vi "FT_sensor_tester old.vi"() -> ()   [LabVIEW 2018]
uses:
  <vilib>/Analysis/baseanly.llb/A x Vector.vi
  <vilib>/Analysis/NI_AALBase.lvlib
panel:
  out "Array":T1(array[cluster])
  out "x-y":u16
  out "Calibrated":dbl[](array[numeric]) format="%.2f"
  in  "Stop Acquisition":bool
  in  "Start Acquisition":bool
  in  "Get Sensor Buffer":bool
  out "Sensor Data":T2
  out "System Status":cluster{"boardState":u8}
  in  "Get Sensor Data":bool
  out "Error Code":T3(ring)
  out "Return FID":u8=2
  out "FID":u8=2
  in  "IP Address":string="192.168.5.001"
  out "System Info":T4
  out "error out":errorcluster
  in  "Get System Info":bool
  in  "Get System Status":bool
  in  "Stop":bool
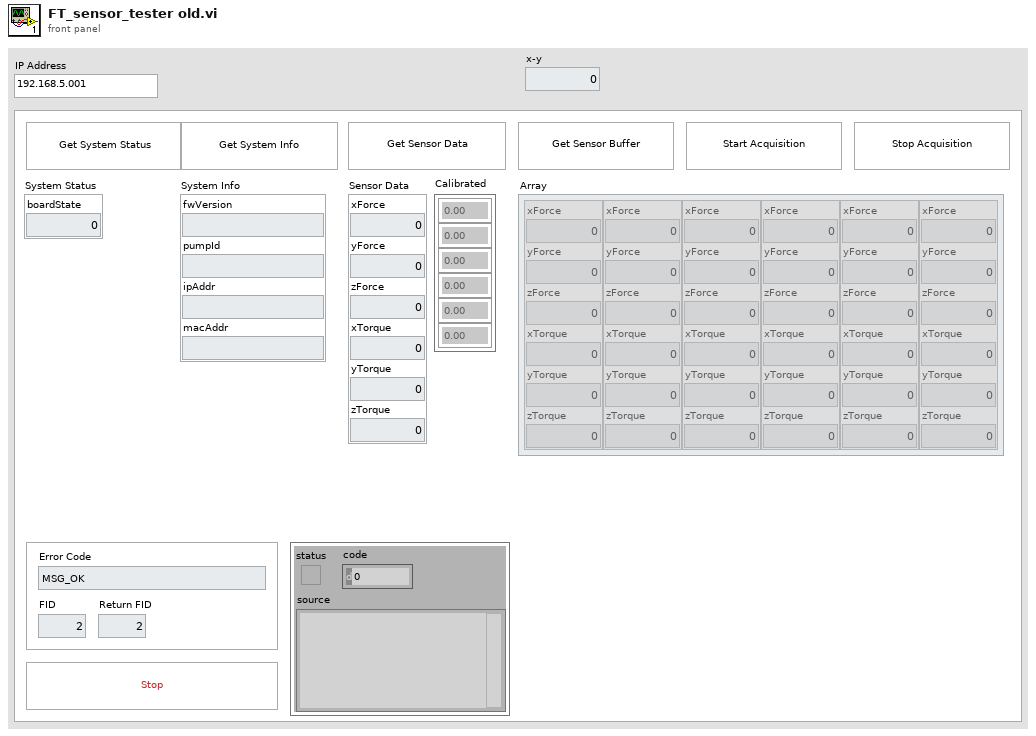
[diagram p1: front panel]
types:
  T1 = cluster{"xForce":sgl, "yForce":sgl, "zForce":sgl, "xTorque":sgl, "yTorque":sgl, "zTorque":sgl}[]
  T2 = cluster{"xForce":sgl, "yForce":sgl, "zForce":sgl, "xTorque":sgl, "yTorque":sgl, "zTorque":sgl}
  T3 = enum8{"MSG_OK", "MSG_ERROR_NOT_SUPPORTED", "MSG_ERROR_SENSOR_DISCONNECTED", "MSG_ERROR_READING_PENDING"}
  T4 = cluster{"fwVersion":string, "pumpId":string, "ipAddr":string, "macAddr":string}
  T5 = cluster{"fwVersion":string, "pumpId":string, "macAddr":string, "ipAddr":string}
  T6 = enum16{"big-endian, network order", "native, host order", "little-endian"}
  T7 = cluster{"pumpState":i32, "suppliedVolume_ml":sgl, "flowRate_mlmin":sgl, "home":i32, "port":i32}
  T8 = cluster{"connection ID":refnum<k5>, "header length":u16}
  T9 = cluster{"boardState":u8, "tempSetpoint":sgl, "pH connected":bool, "Temp connected":bool, "pidOutput":dbl, "pidIntegral":dbl, "pidSetpoint":sgl, "pidStep":sgl, "pidMethod":u8}
  T10 = cluster{"header":cluster{"length":u16, "fid":u8, "error":u8}}
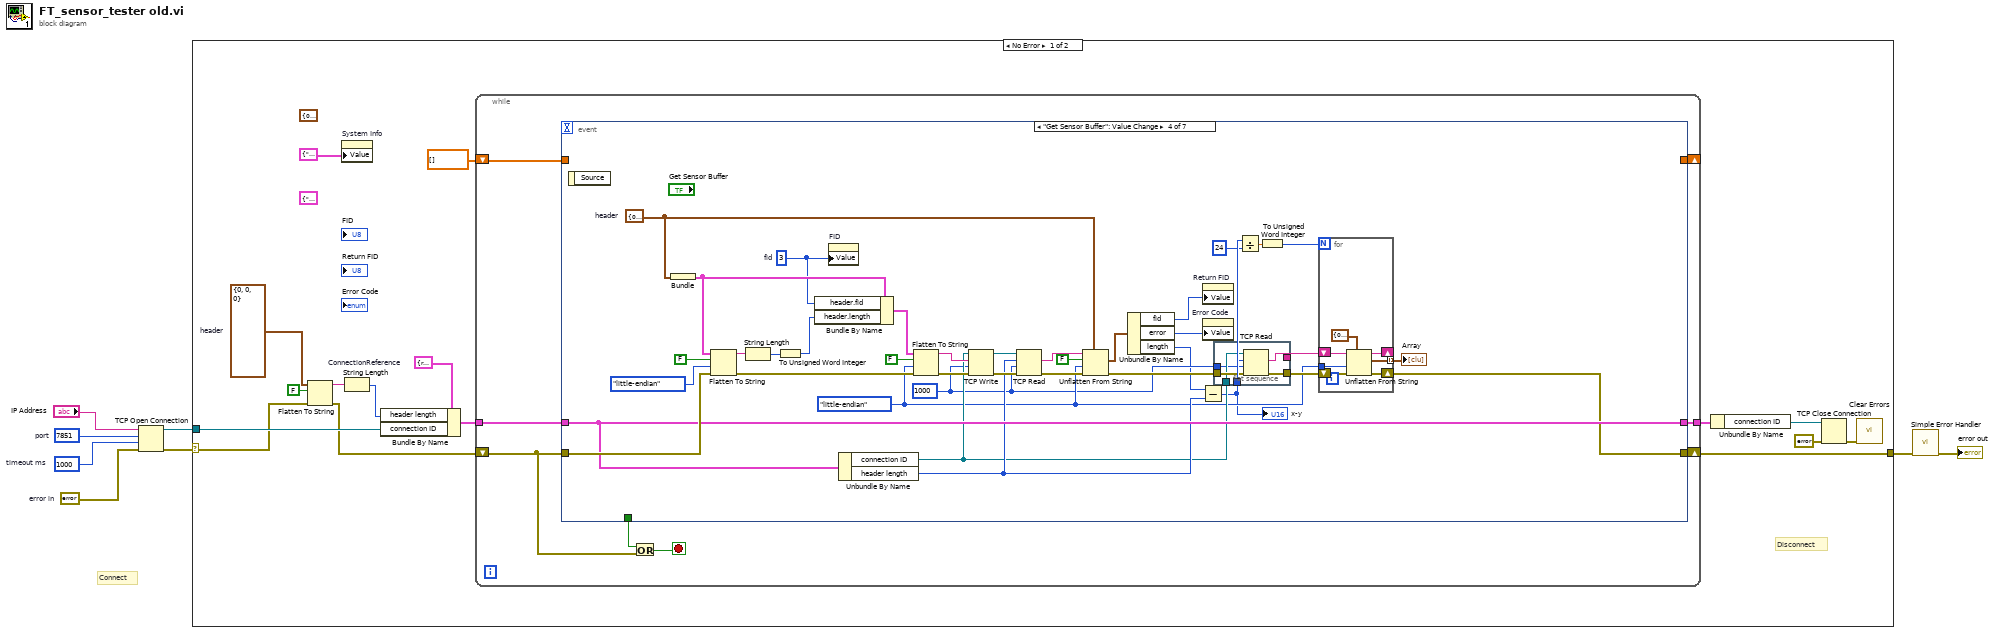
[diagram p0: block diagram]
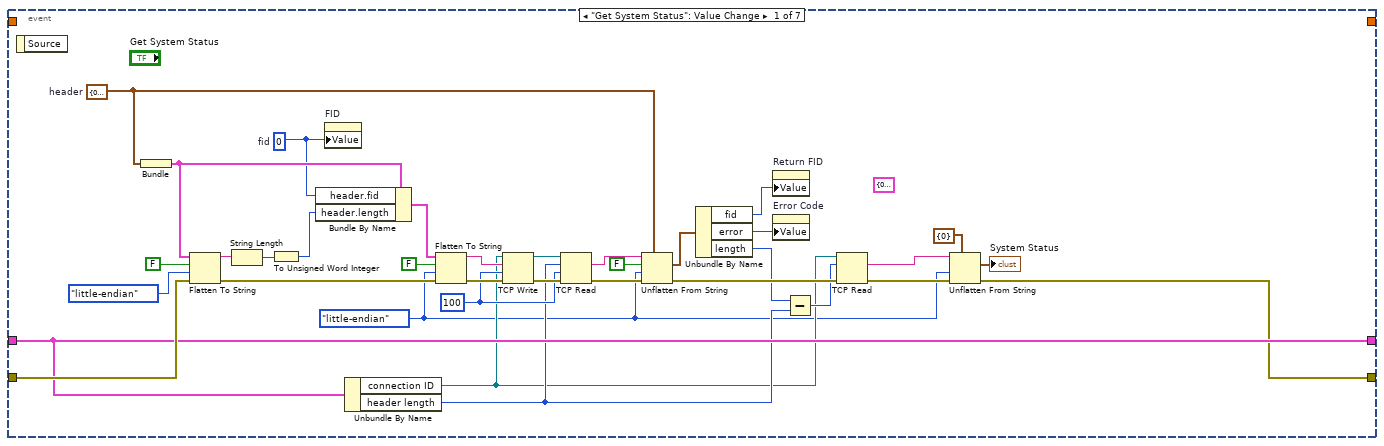
[diagram p2: hidden frame]
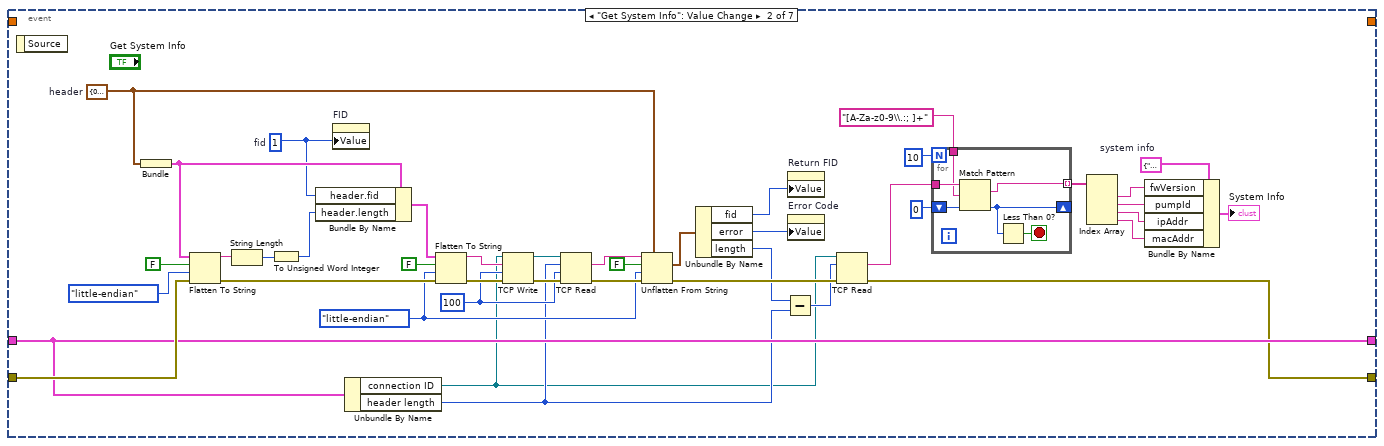
[diagram p3: hidden frame]
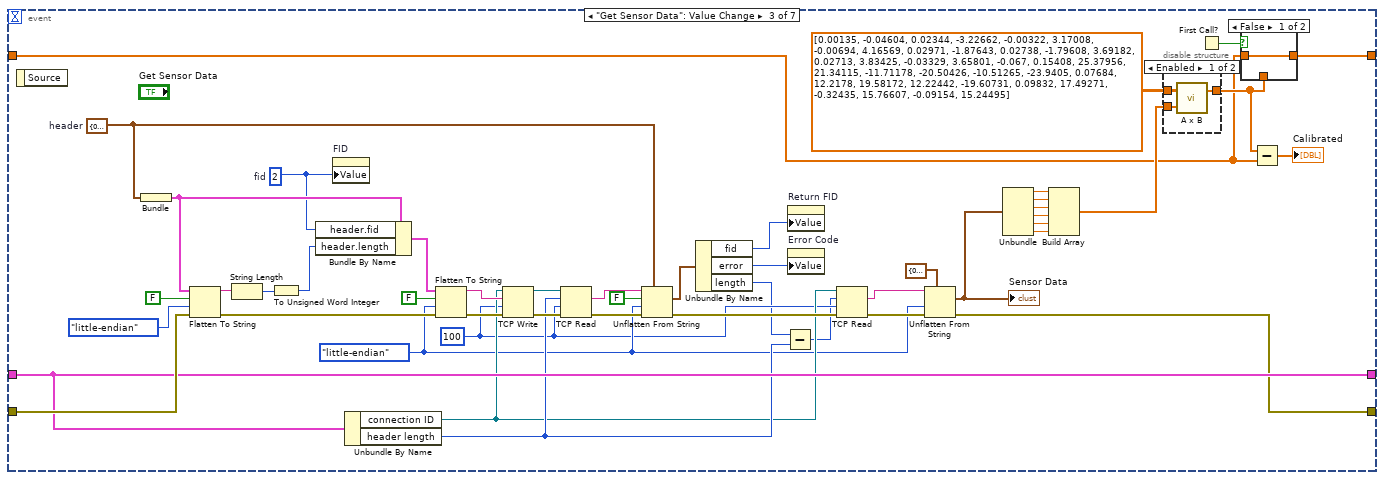
[diagram p4: hidden frame]
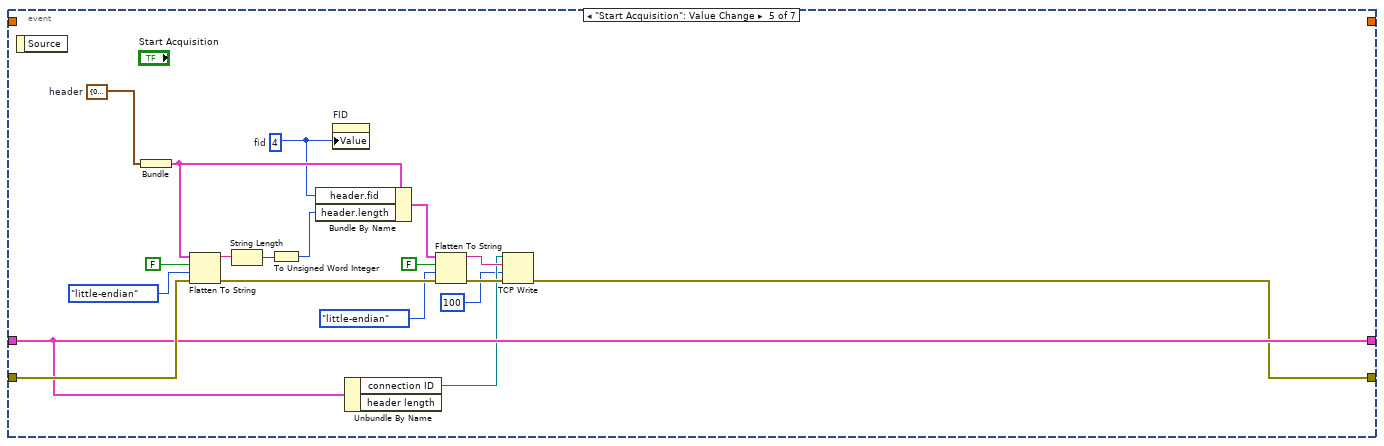
[diagram p7: hidden frame]
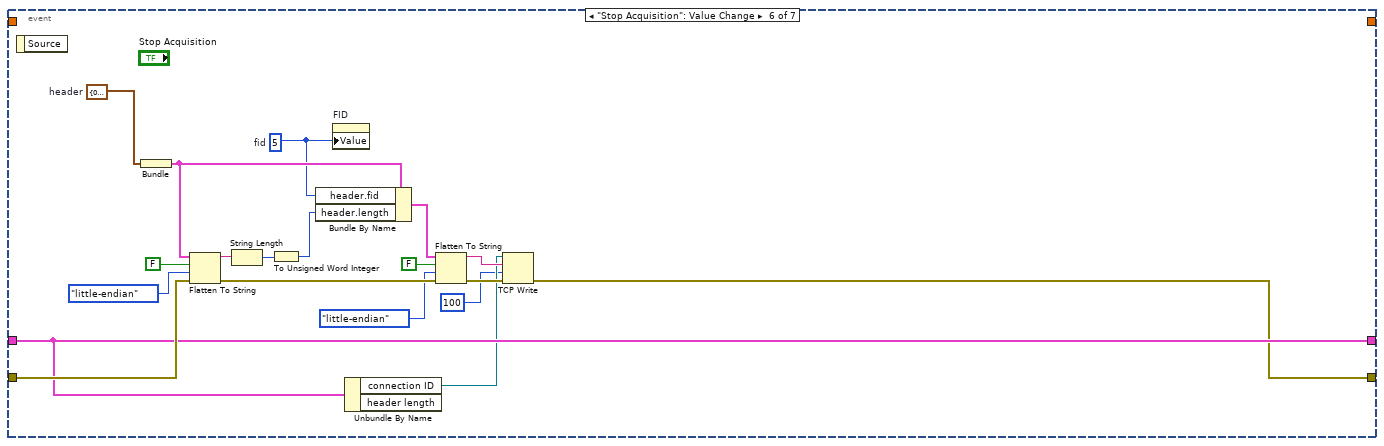
[diagram p8: hidden frame]
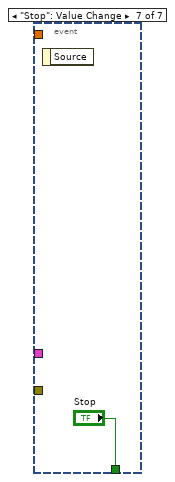
[diagram p9: hidden frame]
diagram:
  w6 = errorcluster {"status"=FALSE, "code"=0, "source"=""}  # error in
  w7 = 1000  # timeout ms
  w8 = u16 7851  # port
  # "Connect"
  n1 = TCP Open Connection(address="IP Address", remote port or service name=w8, timeout ms (60000)=w7, error in (no error)=w6) -> (connection ID=w5:refnum<k5>, error out=w1:errorcluster)  [unwired: 1 in]
  n2 = case shown="No Error" w1 {
    selector: w1 -> [w11 w259]
    tunnel: w5 -> [w20 _]
    tunnel: [w12 w259] -> w2
    frame No Error {
      (unwired) cluster{"axis":string, "stepPeriod (ms)":string} {"axis"="", "stepPeriod (ms)"=""} ("Return Motor Config")
      (unwired) T7 {"pumpState"=0, "suppliedVolume_ml"=0.0, "flowRate_mlmin"=0.0, "home"=0, "port"=0} ("Status")
      w19 = cluster{"length":u16, "fid":u8, "error":u8} {"length"=0, "fid"=0, "error"=0}  # header
      w21 = T8 {"connection ID"=refnum, "header length"=0}  # ConnectionReference
      # "Disconnect"
      n3 = Flatten To String(anything=w19, prepend array or string size? (T)=FALSE, error in (no error)=w11) -> (data string=w17:string, error out=w13:errorcluster)  [unwired: 1 in, 1 out]
      n4 = property on="System Info" class="Clust (strict)"("Value"=T5 {"fwVersion"="", "pumpId"="", "macAddr"="", "ipAddr"=""} ("system info")) -> ()  [unwired: 2 in, 2 out]
      n5 = String Length(string=w17) -> (length=w16:i32)
      n6 = Bundle By Name(cluster=w21, "header length"=w16, "connection ID"=w20) -> (w15:T8)
      n7 = while {
        tunnel: w15 -> [w32]
        tunnel: [w31] -> w14
        shift-right: [w30] -> w12
        shift-left: w13 -> [w28]
        shift-right: [w26] -> _
        shift-left: dbl[] [] ("A x Vector") -> [w25]
        stop <- w29 stop-if-true
        n8 = event shown="[3] \"Get Sensor Buffer\": Value Change" {
          selector: _ -> [_ _ _ _ _ _ _]
          dyn-events: _ -> [_ _ _ _ _ _ _]
          timeout: _ -> [_ _ _ _ _ _ _]
          tunnel: w32 -> [w56 w98 w152 w195 w227 w246 _]
          tunnel: [w56 w98 w152 w195 w227 w246 _] -> w31
          tunnel: w28 -> [w57 w99 w153 w196 w228 w247 _]
          tunnel: [w39 w75 w136 w179 w220 w239 _] -> w30
          tunnel: [_ _ _ _ _ _ "Stop"] -> w27
          tunnel: [_ _ w119 _ _ _ _] -> w26
          tunnel: w25 -> [_ _ w117 _ _ _ _]
          event "Get System Status": Value Change {
            (unwired) T9 {"boardState"=0, "tempSetpoint"=0.0, "pH connected"=FALSE, "Temp connected"=FALSE, "pidOutput"=0.0, "pidIntegral"=0.0, "pidSetpoint"=0.0, "pidStep"=0.0, "pidMethod"=0} ("Status")
            w48 = cluster{"length":u16, "fid":u8, "error":u8} {"length"=0, "fid"=0, "error"=0}  # header
            w50 = 100 ("timeout ms (25000)")
            w36 = u8 0  # fid
            w38 = T6."little-endian" ("byte order (0:big-endian, network order)")
            n9 = event-data() -> ()  [unwired: 1 in, 1 out]
            n10 = Bundle("header"=w48) -> (w63:T10)  [unwired: 1 in]
            n11 = Flatten To String(anything=w63, prepend array or string size? (T)=FALSE, byte order (0:big-endian, network order)=T6."little-endian", error in (no error)=w57) -> (data string=w61:string, error out=w62:errorcluster)  [unwired: 1 out]
            n12 = String Length(string=w61) -> (length=w60:i32)
            n13 = To Unsigned Word Integer(number=w60) -> (unsigned 16bit integer=w59:u16)
            n14 = Bundle By Name(cluster=w63, "header.fid"=w36, "header.length"=w59) -> (w64:T10)
            n15 = property on="FID" class="DigNum (strict)"("Value"=w36) -> ()  [unwired: 2 in, 2 out]
            n16 = Unbundle By Name(w56) -> ("connection ID"=w42:refnum<k5>, "header length"=w44:u16)
            n17 = Flatten To String(anything=w64, prepend array or string size? (T)=FALSE, byte order (0:big-endian, network order)=w38, error in (no error)=w62) -> (data string=w66:string, error out=w67:errorcluster)  [unwired: 1 out]
            n18 = TCP Write(connection ID=w42, data in=w66, error in (no error)=w67, 9:w50) -> (connection ID out=w51:refnum<k5>, error out=w52:errorcluster)  [unwired: 1 out]
            n19 = TCP Read(connection ID=w51, bytes to read=w44, error in (no error)=w52, 9:w50) -> (data out=w53:string, error out=w54:errorcluster)  [unwired: 1 in, 1 out]
            n20 = Unflatten From String(type=w48, binary string=w53, data includes array or string size? (T)=FALSE, byte order (0:big-endian, network order)=w38, error in (no error)=w54) -> (value=w49:cluster{"length":u16, "fid":u8, "error":u8}, error out=w46:errorcluster)  [unwired: 1 out]
            n21 = Unbundle By Name(w49) -> ("fid"=w37:u8, "error"=w35:u8, "length"=w45:u16)
            n22 = property on="Return FID" class="DigNum (strict)"("Value"=w37) -> ()  [unwired: 2 in, 2 out]
            n23 = property on="Error Code" class="Enum (strict)"("Value"=w35) -> ()  [unwired: 2 in, 2 out]
            n24 = Subtract(x=w45, y=w44) -> (x-y=w43:u16)
            n25 = TCP Read(connection ID=w42, bytes to read=w43, error in (no error)=w46) -> (data out=w41:string, error out=w40:errorcluster)  [unwired: 2 in, 1 out]
            n26 = Unflatten From String(type=cluster{"boardState":u8} {"boardState"=0} ("System Status"), binary string=w41, byte order (0:big-endian, network order)=w38, error in (no error)=w40) -> (value=→"System Status":cluster{"boardState":u8}, error out=w39:errorcluster)  [unwired: 1 in, 1 out]
          }
          event "Get System Info": Value Change {
            w87 = T4 {"fwVersion"="", "pumpId"="", "ipAddr"="", "macAddr"=""}  # system info
            w89 = cluster{"length":u16, "fid":u8, "error":u8} {"length"=0, "fid"=0, "error"=0}  # header
            w92 = 100 ("timeout ms (25000)")
            w70 = u8 1  # fid
            w91 = T6."little-endian" ("byte order (0:big-endian, network order)")
            n27 = event-data() -> ()  [unwired: 1 in, 1 out]
            n28 = Bundle("header"=w89) -> (w105:T10)  [unwired: 1 in]
            n29 = Flatten To String(anything=w105, prepend array or string size? (T)=FALSE, byte order (0:big-endian, network order)=T6."little-endian", error in (no error)=w99) -> (data string=w103:string, error out=w104:errorcluster)  [unwired: 1 out]
            n30 = String Length(string=w103) -> (length=w102:i32)
            n31 = To Unsigned Word Integer(number=w102) -> (unsigned 16bit integer=w101:u16)
            n32 = Bundle By Name(cluster=w105, "header.fid"=w70, "header.length"=w101) -> (w106:T10)
            n33 = property on="FID" class="DigNum (strict)"("Value"=w70) -> ()  [unwired: 2 in, 2 out]
            n34 = Unbundle By Name(w98) -> ("connection ID"=w71:refnum<k5>, "header length"=w73:u16)
            n35 = Flatten To String(anything=w106, prepend array or string size? (T)=FALSE, byte order (0:big-endian, network order)=w91, error in (no error)=w104) -> (data string=w108:string, error out=w109:errorcluster)  [unwired: 1 out]
            n36 = TCP Write(connection ID=w71, data in=w108, error in (no error)=w109, 9:w92) -> (connection ID out=w93:refnum<k5>, error out=w94:errorcluster)  [unwired: 1 out]
            n37 = TCP Read(connection ID=w93, bytes to read=w73, error in (no error)=w94, 9:w92) -> (data out=w95:string, error out=w96:errorcluster)  [unwired: 1 in, 1 out]
            n38 = Unflatten From String(type=w89, binary string=w95, data includes array or string size? (T)=FALSE, byte order (0:big-endian, network order)=w91, error in (no error)=w96) -> (value=w90:cluster{"length":u16, "fid":u8, "error":u8}, error out=w77:errorcluster)  [unwired: 1 out]
            n39 = Unbundle By Name(w90) -> ("fid"=w69:u8, "error"=w68:u8, "length"=w74:u16)
            n40 = Subtract(x=w74, y=w73) -> (x-y=w72:u16)
            n41 = property on="Return FID" class="DigNum (strict)"("Value"=w69) -> ()  [unwired: 2 in, 2 out]
            n42 = property on="Error Code" class="Enum (strict)"("Value"=w68) -> ()  [unwired: 2 in, 2 out]
            n43 = TCP Read(connection ID=w71, bytes to read=w72, error in (no error)=w77) -> (data out=w85:string, error out=w75:errorcluster)  [unwired: 2 in, 1 out]
            n44 = for {
              N: 10 -> [_]
              shift-right: [w111] -> _
              shift-left: 0 ("offset past match") -> [w115]
              tunnel: w85 -> [w114]
              tunnel: "[A-Za-z0-9\\.:; ]+" ("regular expression") -> [w113]
              tunnel: [w110] -> w82 mode=indexing
              stop <- w112 stop-if-true
              n45 = Match Pattern(string=w114, regular expression=w113, offset (0)=w115) -> (match substring=w110:string, offset past match=w111:i32)  [unwired: 2 out]
              n46 = Less Than 0?(x=w111) -> (x < 0?=w112:bool)
            }
            n47 = Index Array(array=w82) -> (element #1=w81:string, element #2=w80:string, element #3=w79:string, element #4=w78:string)  [unwired: 4 in]
            n48 = Bundle By Name(cluster=w87, "fwVersion"=w81, "pumpId"=w80, "ipAddr"=w79, "macAddr"=w78) -> (→"System Info":T4)
          }
          event "Get Sensor Data": Value Change {
            w145 = cluster{"length":u16, "fid":u8, "error":u8} {"length"=0, "fid"=0, "error"=0}  # header
            w133 = 100 ("timeout ms (25000)")
            w140 = u8 2  # fid
            w134 = T6."little-endian" ("byte order (0:big-endian, network order)")
            n49 = event-data() -> ()  [unwired: 1 in, 1 out]
            n50 = Bundle("header"=w145) -> (w159:T10)  [unwired: 1 in]
            n51 = Flatten To String(anything=w159, prepend array or string size? (T)=FALSE, byte order (0:big-endian, network order)=T6."little-endian", error in (no error)=w153) -> (data string=w157:string, error out=w158:errorcluster)  [unwired: 1 out]
            n52 = String Length(string=w157) -> (length=w156:i32)
            n53 = To Unsigned Word Integer(number=w156) -> (unsigned 16bit integer=w155:u16)
            n54 = Bundle By Name(cluster=w159, "header.fid"=w140, "header.length"=w155) -> (w160:T10)
            n55 = property on="FID" class="DigNum (strict)"("Value"=w140) -> ()  [unwired: 2 in, 2 out]
            n56 = Unbundle By Name(w152) -> ("connection ID"=w141:refnum<k5>, "header length"=w142:u16)
            n57 = Flatten To String(anything=w160, prepend array or string size? (T)=FALSE, byte order (0:big-endian, network order)=w134, error in (no error)=w158) -> (data string=w162:string, error out=w163:errorcluster)  [unwired: 1 out]
            n58 = TCP Write(connection ID=w141, data in=w162, error in (no error)=w163, 9:w133) -> (connection ID out=w147:refnum<k5>, error out=w148:errorcluster)  [unwired: 1 out]
            n59 = TCP Read(connection ID=w147, bytes to read=w142, error in (no error)=w148, 9:w133) -> (data out=w149:string, error out=w150:errorcluster)  [unwired: 1 in, 1 out]
            n60 = Unflatten From String(type=w145, binary string=w149, data includes array or string size? (T)=FALSE, byte order (0:big-endian, network order)=w134, error in (no error)=w150) -> (value=w146:cluster{"length":u16, "fid":u8, "error":u8}, error out=w143:errorcluster)  [unwired: 1 out]
            n61 = Unbundle By Name(w146) -> ("fid"=w139:u8, "error"=w138:u8, "length"=w130:u16)
            n62 = Subtract(x=w130, y=w142) -> (x-y=w131:u16)
            n63 = property on="Return FID" class="DigNum (strict)"("Value"=w139) -> ()  [unwired: 2 in, 2 out]
            n64 = property on="Error Code" class="Enum (strict)"("Value"=w138) -> ()  [unwired: 2 in, 2 out]
            n65 = TCP Read(connection ID=w141, bytes to read=w131, error in (no error)=w143, 9:w133) -> (data out=w135:string, error out=w137:errorcluster)  [unwired: 1 in, 1 out]
            n66 = Unflatten From String(type=T2 {"xForce"=0.0, "yForce"=0.0, "zForce"=0.0, "xTorque"=0.0, "yTorque"=0.0, "zTorque"=0.0} ("Sensor Data"), binary string=w135, byte order (0:big-endian, network order)=w134, error in (no error)=w137) -> (value=w128:T2, error out=w136:errorcluster)  [unwired: 1 in, 1 out]
            "Sensor Data" <- w128
            n67 = Unbundle(w128) -> ("xForce"=w127:sgl, "yForce"=w122:sgl, "zForce"=w123:sgl, "xTorque"=w124:sgl, "yTorque"=w125:sgl, "zTorque"=w126:sgl)
            n68 = Build Array(w127, w122, w123, w124, w125, w126) -> (w121:sgl[])
            n69 = disable-structure shown="Enabled" {
              disable-tunnel: dbl[][] [[0.00135, -0.04604, 0.02344, -3.22662, -0.00322, 3.17008], [-0.00694, 4.16569, 0.02971, -1.87643, 0.02738, -1.79608], [3.69182, 0.02713, 3.83425, -0.03329, 3.65801, -0.067], [0.15408, 25.37956, 21.34115, -11.71178, -20.50426, -10.51265], [-23.9405, 0.07684, 12.2178, 19.58172, 12.22442, -19.60731], [0.09832, 17.49271, -0.32435, 15.76607, -0.09154, 15.24495]] ("Calibration Matrix") -> [w166 _]
              disable-tunnel: w121 -> [w165 w167]
              disable-tunnel: [w164 w167] -> w118
              frame Enabled {
                n70 = call-poly <vilib>:"A x B.vi"("Vector"=w165, "A"=w166) -> ("A x Vector"=w164:dbl[])  [unwired: 1 out]
              }
              frame Disabled {
              }
            }
            n71 = First Call?() -> (First Call?: T/F=w116:bool)
            n72 = case shown="False" w116 {
              tunnel: [w168 w169] -> w119
              tunnel: w118 -> [_ w169]
              tunnel: w117 -> [w168 _]
              frame False {
              }
              frame True {
              }
            }
            n73 = Subtract(x=w118, y=w117) -> (x-y=→"Calibrated":dbl[])
          }
          event "Get Sensor Buffer": Value Change {
            w188 = cluster{"length":u16, "fid":u8, "error":u8} {"length"=0, "fid"=0, "error"=0}  # header
            w177 = 1000 ("timeout ms (25000)")
            w183 = u8 3  # fid
            w178 = T6."little-endian" ("byte order (0:big-endian, network order)")
            n74 = event-data() -> ()  [unwired: 1 in, 1 out]
            n75 = Bundle("header"=w188) -> (w202:T10)  [unwired: 1 in]
            n76 = Flatten To String(anything=w202, prepend array or string size? (T)=FALSE, byte order (0:big-endian, network order)=T6."little-endian", error in (no error)=w196) -> (data string=w200:string, error out=w201:errorcluster)  [unwired: 1 out]
            n77 = String Length(string=w200) -> (length=w199:i32)
            n78 = To Unsigned Word Integer(number=w199) -> (unsigned 16bit integer=w198:u16)
            n79 = Bundle By Name(cluster=w202, "header.fid"=w183, "header.length"=w198) -> (w203:T10)
            n80 = property on="FID" class="DigNum (strict)"("Value"=w183) -> ()  [unwired: 2 in, 2 out]
            n81 = Unbundle By Name(w195) -> ("connection ID"=w184:refnum<k5>, "header length"=w185:u16)
            n82 = Flatten To String(anything=w203, prepend array or string size? (T)=FALSE, byte order (0:big-endian, network order)=w178, error in (no error)=w201) -> (data string=w205:string, error out=w206:errorcluster)  [unwired: 1 out]
            n83 = TCP Write(connection ID=w184, data in=w205, error in (no error)=w206, 9:w177) -> (connection ID out=w190:refnum<k5>, error out=w191:errorcluster)  [unwired: 1 out]
            n84 = TCP Read(connection ID=w190, bytes to read=w185, error in (no error)=w191, 9:w177) -> (data out=w192:string, error out=w193:errorcluster)  [unwired: 1 in, 1 out]
            n85 = Unflatten From String(type=w188, binary string=w192, data includes array or string size? (T)=FALSE, byte order (0:big-endian, network order)=w178, error in (no error)=w193) -> (value=w189:cluster{"length":u16, "fid":u8, "error":u8}, error out=w186:errorcluster)  [unwired: 1 out]
            n86 = Unbundle By Name(w189) -> ("fid"=w182:u8, "error"=w181:u8, "length"=w176:u16)
            n87 = Subtract(x=w176, y=w185) -> (x-y=w175:u16)
            "x-y" <- w175
            n88 = property on="Return FID" class="DigNum (strict)"("Value"=w182) -> ()  [unwired: 2 in, 2 out]
            n89 = property on="Error Code" class="Enum (strict)"("Value"=w181) -> ()  [unwired: 2 in, 2 out]
            n90 = flat-sequence {
              tunnel: w186 -> [w212]
              tunnel: w184 -> [w211]
              tunnel: [w210] -> w180
              tunnel: [w209] -> w171
              tunnel: w177 -> [w208]
              tunnel: w175 -> [w207]
              frame #0 {
                n91 = TCP Read(connection ID=w211, bytes to read=w207, error in (no error)=w212, 9:w208) -> (data out=w209:string, error out=w210:errorcluster)  [unwired: 1 in, 1 out]
              }
            }
            n92 = Divide(x=w175, y=u16 24) -> (x/y=w173:dbl)
            n93 = To Unsigned Word Integer(number=w173) -> (unsigned 16bit integer=w172:u16)
            n94 = for {
              N: w172 -> [_]
              tunnel: w178 -> [w216]
              shift-right: [w218] -> w179
              shift-left: w180 -> [w219]
              tunnel: [w215] -> w170 mode=indexing
              shift-right: [w214] -> _
              shift-left: w171 -> [w217]
              n95 = Unflatten From String(type=T2 {"xForce"=0.0, "yForce"=0.0, "zForce"=0.0, "xTorque"=0.0, "yTorque"=0.0, "zTorque"=0.0} ("Sensor Data"), binary string=w217, byte order (0:big-endian, network order)=w216, error in (no error)=w219) -> (rest of the binary string=w214:string, value=w215:T2, error out=w218:errorcluster)  [unwired: 1 in]
            }
            "Array" <- w170
          }
          event "Start Acquisition": Value Change {
            w226 = cluster{"length":u16, "fid":u8, "error":u8} {"length"=0, "fid"=0, "error"=0}  # header
            w223 = u8 4  # fid
            n96 = event-data() -> ()  [unwired: 1 in, 1 out]
            n97 = Bundle("header"=w226) -> (w234:T10)  [unwired: 1 in]
            n98 = Flatten To String(anything=w234, prepend array or string size? (T)=FALSE, byte order (0:big-endian, network order)=T6."little-endian", error in (no error)=w228) -> (data string=w232:string, error out=w233:errorcluster)  [unwired: 1 out]
            n99 = String Length(string=w232) -> (length=w231:i32)
            n100 = To Unsigned Word Integer(number=w231) -> (unsigned 16bit integer=w230:u16)
            n101 = Bundle By Name(cluster=w234, "header.fid"=w223, "header.length"=w230) -> (w235:T10)
            n102 = property on="FID" class="DigNum (strict)"("Value"=w223) -> ()  [unwired: 2 in, 2 out]
            n103 = Unbundle By Name(w227) -> ("connection ID"=w224:refnum<k5>)  [unwired: 1 out]
            n104 = Flatten To String(anything=w235, prepend array or string size? (T)=FALSE, byte order (0:big-endian, network order)=T6."little-endian", error in (no error)=w233) -> (data string=w237:string, error out=w238:errorcluster)  [unwired: 1 out]
            n105 = TCP Write(connection ID=w224, data in=w237, error in (no error)=w238, 9:100 ("timeout ms (25000)")) -> (error out=w220:errorcluster)  [unwired: 2 out]
          }
          event "Stop Acquisition": Value Change {
            w245 = cluster{"length":u16, "fid":u8, "error":u8} {"length"=0, "fid"=0, "error"=0}  # header
            w242 = u8 5  # fid
            n106 = event-data() -> ()  [unwired: 1 in, 1 out]
            n107 = Bundle("header"=w245) -> (w253:T10)  [unwired: 1 in]
            n108 = Flatten To String(anything=w253, prepend array or string size? (T)=FALSE, byte order (0:big-endian, network order)=T6."little-endian", error in (no error)=w247) -> (data string=w251:string, error out=w252:errorcluster)  [unwired: 1 out]
            n109 = String Length(string=w251) -> (length=w250:i32)
            n110 = To Unsigned Word Integer(number=w250) -> (unsigned 16bit integer=w249:u16)
            n111 = Bundle By Name(cluster=w253, "header.fid"=w242, "header.length"=w249) -> (w254:T10)
            n112 = property on="FID" class="DigNum (strict)"("Value"=w242) -> ()  [unwired: 2 in, 2 out]
            n113 = Unbundle By Name(w246) -> ("connection ID"=w243:refnum<k5>)  [unwired: 1 out]
            n114 = Flatten To String(anything=w254, prepend array or string size? (T)=FALSE, byte order (0:big-endian, network order)=T6."little-endian", error in (no error)=w252) -> (data string=w256:string, error out=w257:errorcluster)  [unwired: 1 out]
            n115 = TCP Write(connection ID=w243, data in=w256, error in (no error)=w257, 9:100 ("timeout ms (25000)")) -> (error out=w239:errorcluster)  [unwired: 2 out]
          }
          event "Stop": Value Change {
            n116 = event-data() -> ()  [unwired: 1 in, 1 out]
          }
        }
        n117 = Or(x=w27, y=w28) -> (x .or. y?=w29:bool)
      }
      n118 = Unbundle By Name(w14) -> ("connection ID"=w22:refnum<k5>)
      n119 = TCP Close Connection(connection ID=w22, error in (no error)=errorcluster {"status"=FALSE, "code"=0, "source"=""}) -> (error out=w23:errorcluster)  [unwired: 1 in, 1 out]
      n120 = call <vilib>:"Clear Errors.vi"("error in (no error)"=w23) -> ()  [unwired: 5 in, 2 out]
    }
    frame Error {
    }
  }
  n121 = call <vilib>:"Simple Error Handler.vi"("error in (no error)"=w2) -> ("error out"=→"error out":errorcluster)  [unwired: 4 in, 4 out]
